vi "Dynamixel Motor Record and Playback Motion (Synchronous Write).vi"() -> ()   [LabVIEW 2016]
doc: "This example demonstrates how to capture sets of motor positions (frames) and then play them back. The playback feature also shows how to generate a sychronous write command that sets the goal position and velocity of all of the motors simultaneously."
uses:
  <instrlib>/Dynamixel Motor/Public/Motor Operation/Low Level/Baud Setting.ctl
  <instrlib>/Dynamixel Motor/Examples/Record And Playback Motion/Type Defs/Compiled Motion.ctl
  <instrlib>/Dynamixel Motor/Dynamixel Motor.lvlib
panel:
  in  "Initialize or Go":bool
  in  "Stop Playback":bool
  in  "Delay Time (ms)":dbl
  in  "Speed Scale (%)":dbl=100.0
  in  "Play":bool
  in  "Paste":bool
  in  "Copy":bool
  in  "Delete":bool
  in  "Insert":bool
  in  "Record":bool
  in  "Frame":u16
  in  "Step Time (ms)":u32=600
  in  "Baud rate (57600 bps)":T1=34 items=["1,000,000 bps"=1, "500,000 bps"=3, "400,000 bps"=4, "250,000 bps"=7, "200,000 bps"=9, "115200 bps"=16, "57600 bps"=34, "19200 bps"=103, "9600 bps"=207]
  in  "VISA resource name":refnum<visa-resource-name>
  in  "Up to":u8=253
  in  "From":u8
  in  "Refresh Motor List":bool
  in  "Motor Torques":cluster{"On":bool, "Off":bool, "ID":u8}[](array[cluster])
  in  "Torque off":bool
  in  "Save":bool
  in  "Load":bool
  in  "Quit":bool
  in  "Torque on":bool
  in  "Display Table":string[][](table)
  # "Motor List"
  # "Motor Torques"
  # "Frame number >>"
  # "Shortcuts: \n<Escape>-->Stop Playback\n<Enter>-->Go\n<Page Up>-->All on\n<Page Down>-->All off"
  # "1. Set the serial settings\n2. Run the VI\n3. click  Refresh Motor List to find connected motors.\n3. Click Record to capture the positions of all of the motors.\n4. Move the motors to a different position and click Record again.\n5. Change Frame to 0 or click on the first column of positions, then click Go.  Then Click Play.\n7. For more information and instructions, see the Readme."
  # "(c) 2011-2012  National Instruments.  ALL RIGHTS RESERVED."
  # "Playback"
  # "Record Positions"
  # "Initialization"
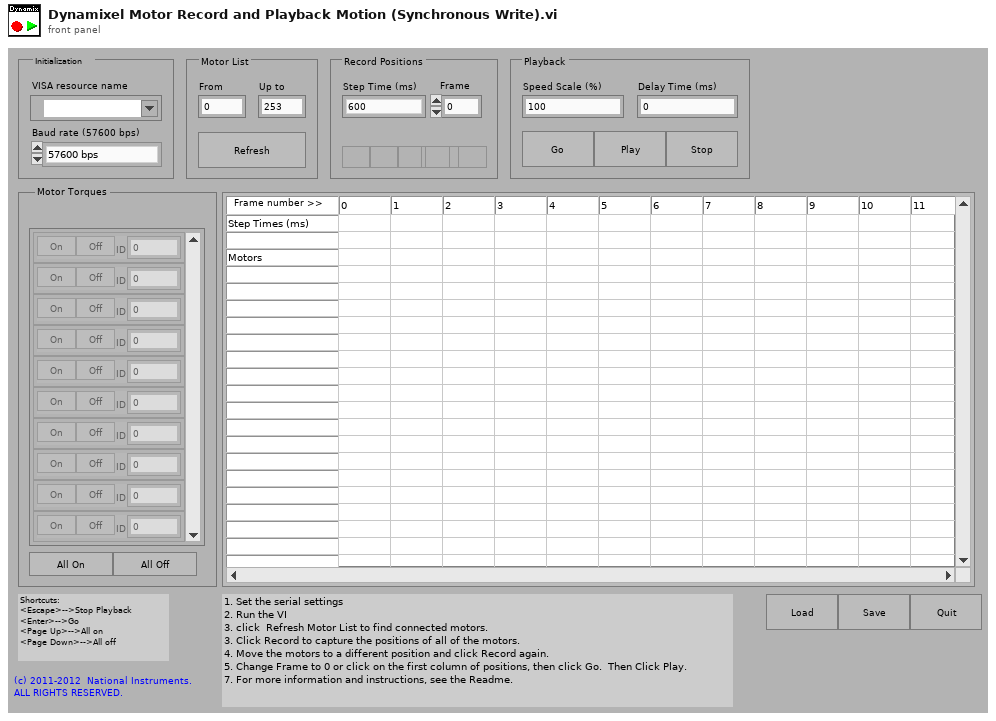
[diagram p1: front panel]
types:
  T1 = typedef "Dynamixel Motor.lvlib/Baud Setting.ctl" = u8
  T2 = typedef "Compiled Motion.ctl" = cluster{"Step Times":dbl[], "Serial Commands":string[], "Title":string}
  T3 = typedef "LVRowAndColumnTypeDef.ctl" = cluster{"Row":i32, "Column":i32}
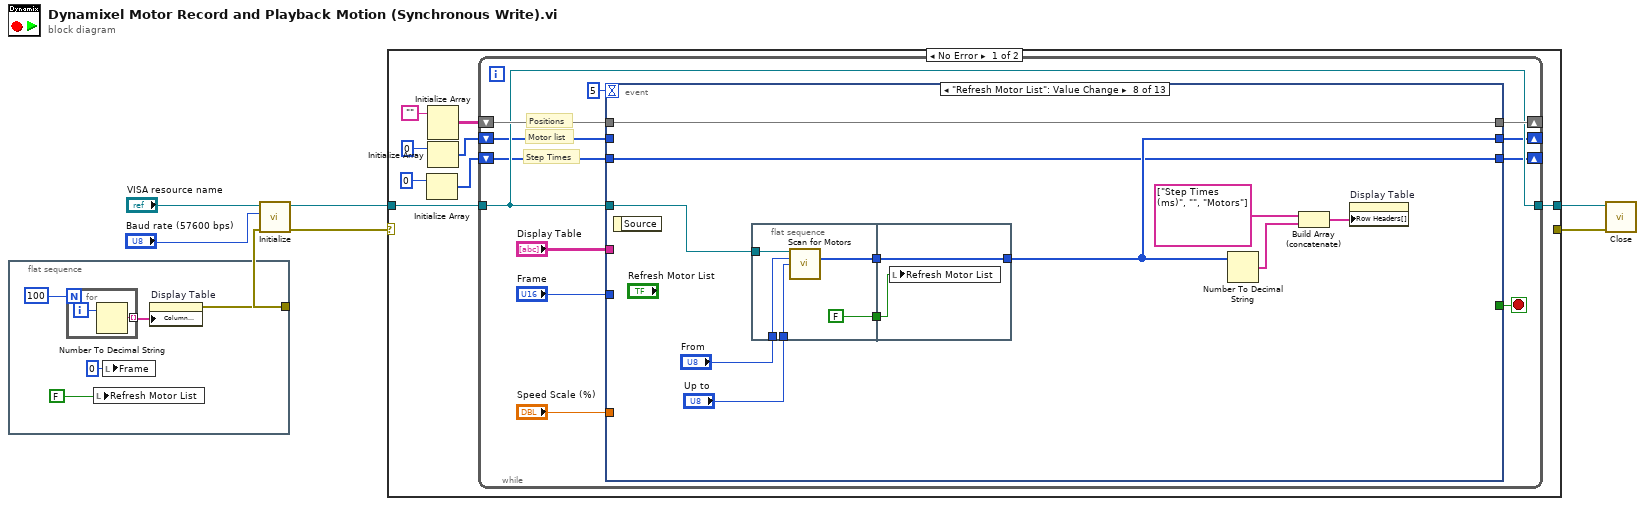
[diagram p0: block diagram]
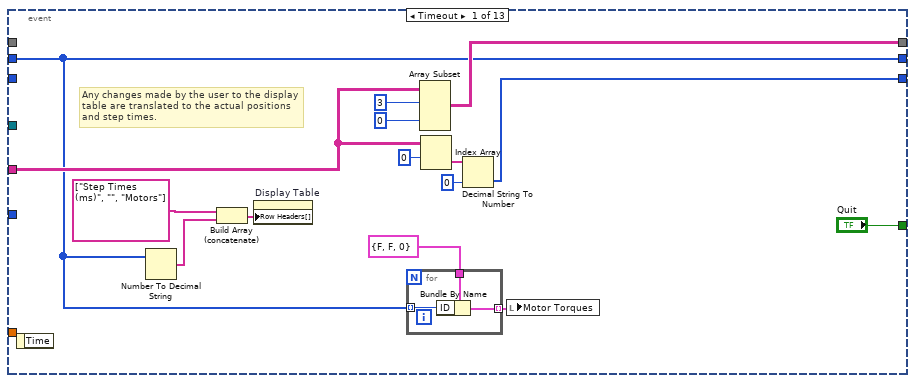
[diagram p2: hidden frame]
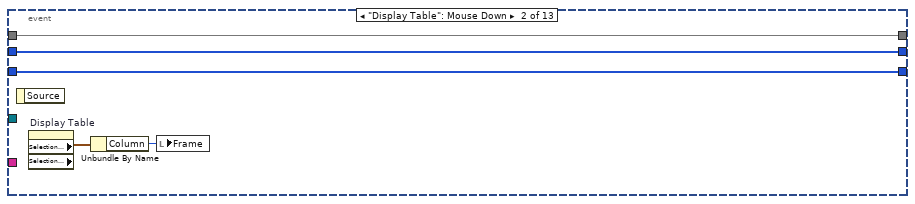
[diagram p3: hidden frame]
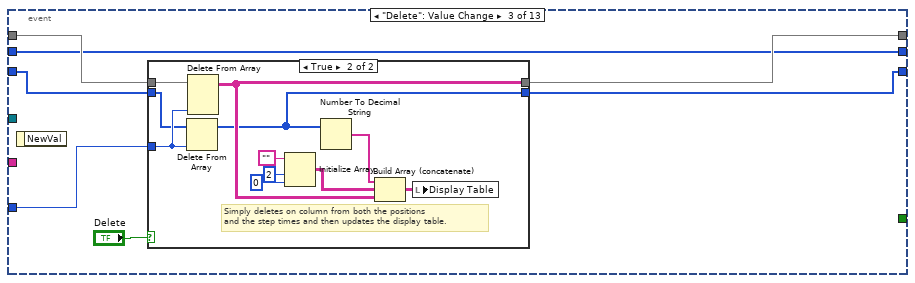
[diagram p4: hidden frame]
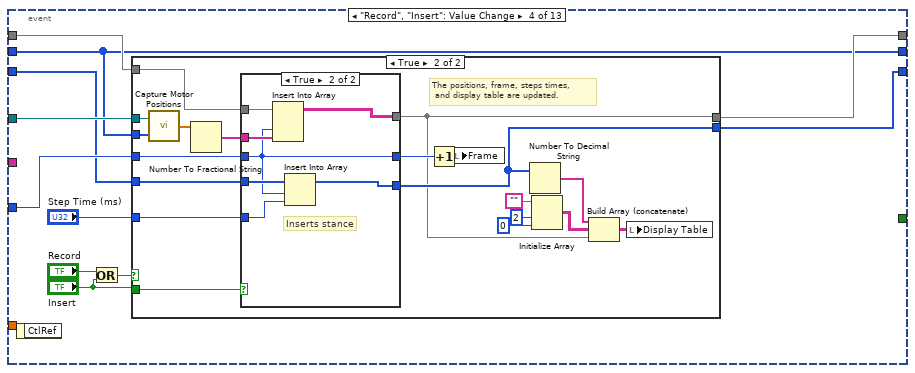
[diagram p6: hidden frame]
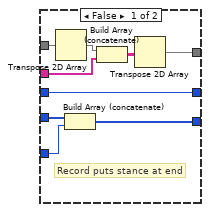
[diagram p8: hidden frame]
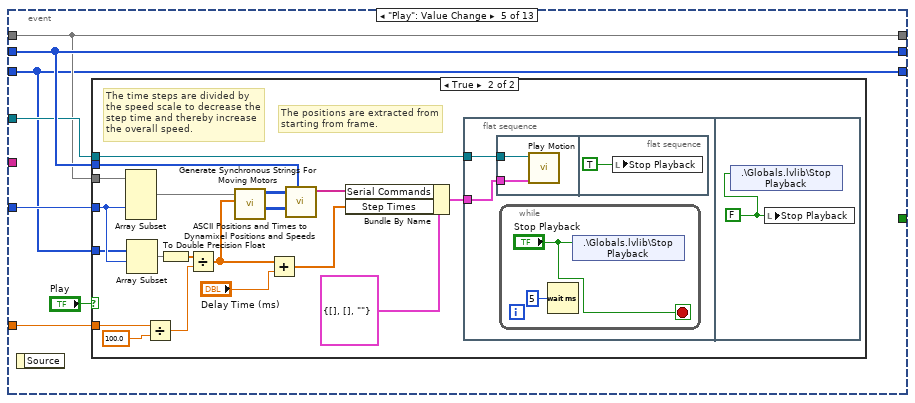
[diagram p9: hidden frame]
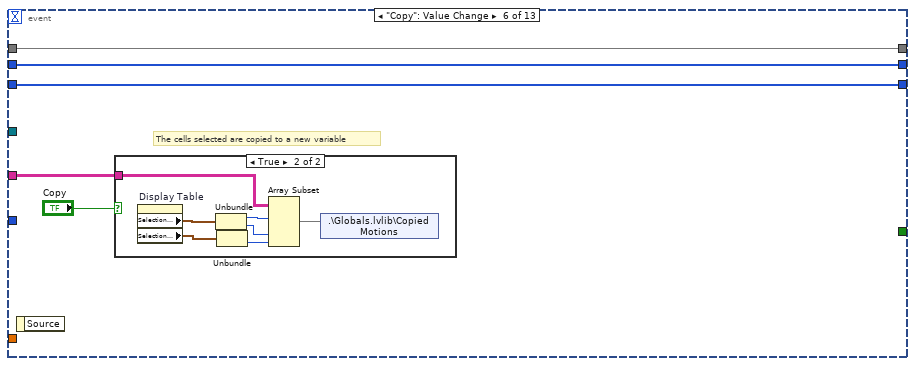
[diagram p11: hidden frame]
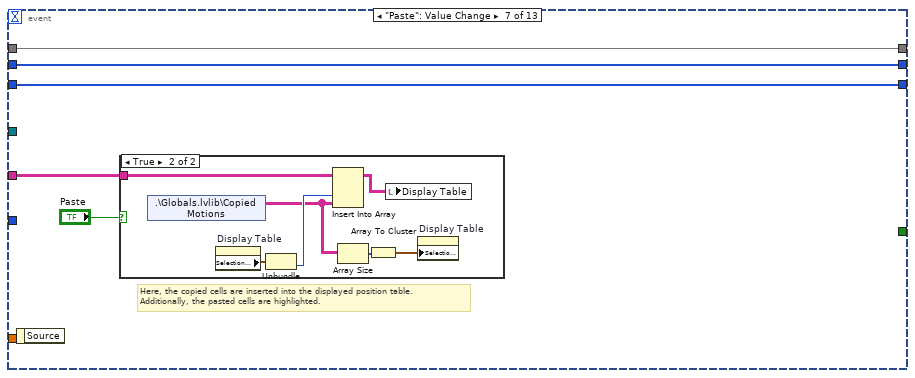
[diagram p13: hidden frame]
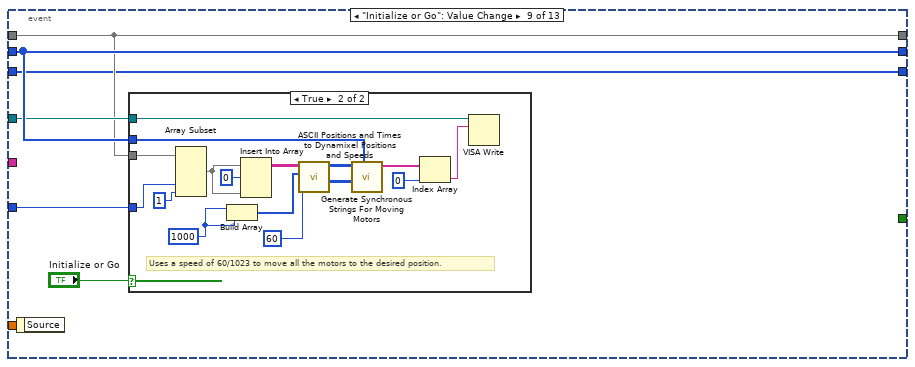
[diagram p15: hidden frame]
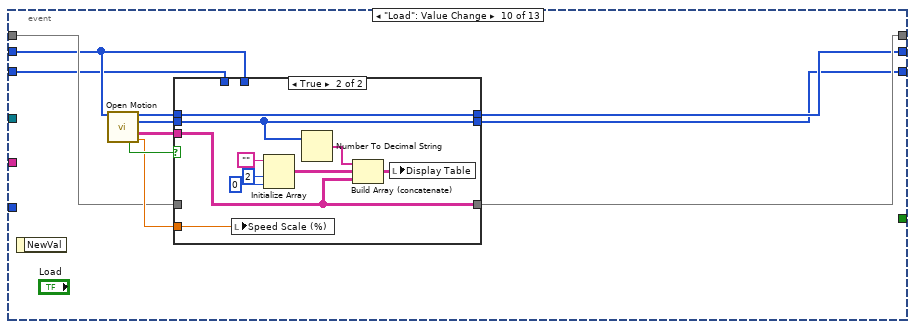
[diagram p17: hidden frame]
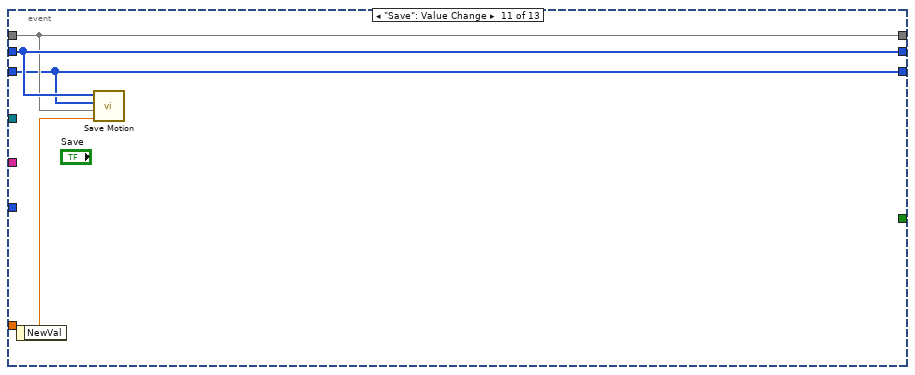
[diagram p19: hidden frame]
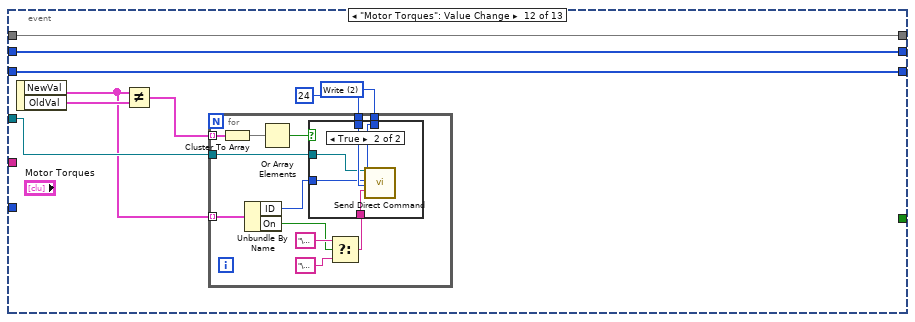
[diagram p20: hidden frame]
diagram:
  n1 = flat-sequence {
    tunnel: [w10] -> w4
    frame #0 {
      n2 = for {
        N: 100 -> [_]
        tunnel: [w13] -> w12 mode=indexing
        i -> [w14]
        n3 = Number To Decimal String(number=w14) -> (decimal integer string=w13:string)  [unwired: 1 in]
      }
      n4 = local write "Refresh Motor List"(FALSE ("Searching...")) -> ()
      n5 = local write "Frame"(u16 0 ("Frame")) -> ()
      n6 = property on="Display Table" class="Tbl (strict)"("Column Headers[]"=w12) -> (error out=w10:errorcluster)  [unwired: 2 in, 1 out]
    }
  }
  n7 = call <instrlib>:"Initialize.vi"("error in (no error)"=w4, "Baud rate (57600 bps)"="Baud rate (57600 bps)", "VISA resource name"="VISA resource name") -> ("error out"=w1:errorcluster, "VISA resource name out"=w7:refnum<visa-resource-name>)  [unwired: 7 in]
  n8 = case shown="No Error" w1 {
    selector: w1 -> [_ w290]
    tunnel: w7 -> [w22 w289]
    tunnel: [_ w290] -> w3
    tunnel: [w19 w289] -> w2
    frame No Error {
      n9 = Initialize Array(u32 0) -> (w15:u32[])  [unwired: 1 in]
      n10 = Initialize Array("") -> (w20:string[][])  [unwired: 2 in]
      n11 = Initialize Array(u8 0) -> (w18:u8[])  [unwired: 1 in]
      n12 = while {
        tunnel: w22 -> [w27]
        shift-right: [w29] -> _
        shift-left: w20 -> [w28]
        tunnel: [w27] -> w19
        shift-right: [w26] -> _
        shift-left: w18 -> [w25]
        shift-right: [w24] -> _
        shift-left: w15 -> [w23]
        stop <- w34 stop-if-true
        # "Step Times"
        # "Motor list"
        # "Positions"
        n13 = event shown="[7] \"Refresh Motor List\": Value Change" {
          selector: _ -> [_ _ _ _ _ _ _ _ _ _ _ _ _]
          dyn-events: _ -> [_ _ _ _ _ _ _ _ _ _ _ _ _]
          timeout: 5 -> [_ _ _ _ _ _ _ _ _ _ _ _ _]
          tunnel: "Frame" -> [_ _ w62 w84 w131 _ _ _ w206 _ _ _ _]
          tunnel: w27 -> [_ _ _ w83 w129 _ _ w191 w204 _ _ w256 w281]
          tunnel: w25 -> [w36 w54 w60 w80 w130 w161 w173 _ w205 w226 w251 w253 w279]
          tunnel: "Display Table" -> [w43 _ _ _ _ w164 w176 _ _ _ _ _ _]
          tunnel: w28 -> [_ w55 w63 w82 w127 w162 w174 w186 w203 w228 w249 w254 w280]
          tunnel: "Speed Scale (%)" -> [_ _ _ _ w128 _ _ _ _ _ w250 _ _]
          tunnel: ["Quit" _ _ _ _ _ _ _ _ _ _ _ _] -> w34
          tunnel: [w37 w55 w61 w81 w127 w162 w174 w186 w203 w229 w249 w254 w280] -> w29
          tunnel: [w36 w54 w60 w80 w130 w161 w173 w185 w205 w227 w251 w253 w279] -> w26
          tunnel: [w35 w53 w59 w79 w126 w160 w172 w184 w202 w225 w248 w252 w278] -> w24
          tunnel: w23 -> [_ w53 w58 w78 w126 w160 w172 w184 w202 w224 w248 w252 w278]
          event Timeout {
            # "Any changes made by the user to the display \ntable are translated to the actual positions \nand step times."
            n14 = event-data() -> ()  [unwired: 1 in, 1 out]
            n15 = Number To Decimal String(number=w36) -> (decimal integer string=w47:string[])  [unwired: 1 in]
            n16 = Build Array (concatenate)(string[] ["Step Times (ms)", "", "Motors"], w47) -> (w46:string[])
            n17 = property on="Display Table" class="Tbl (strict)"("Row Headers[]"=w46) -> ()  [unwired: 2 in, 2 out]
            n18 = for {
              tunnel: w36 -> [w52] mode=indexing
              tunnel: cluster{"On":bool, "Off":bool, "ID":u8} {"On"=FALSE, "Off"=FALSE, "ID"=0} ("Cluster") -> [w51]
              tunnel: [w50] -> w39 mode=indexing
              n19 = Bundle By Name(cluster=w51, "ID"=w52) -> (w50:cluster{"On":bool, "Off":bool, "ID":u8})
            }
            n20 = Array Subset(array=w43, index (row)=3 ("index"), index (col)=0 ("index")) -> (w37:string[][])  [unwired: 2 in]
            n21 = Index Array(array=w43, index (row)=0) -> (element=w42:string[])  [unwired: 1 in]
            n22 = Decimal String To Number(string=w42, default (0L)=u32 0 ("default (0 I32)")) -> (number=w35:u32[])  [unwired: 1 in, 1 out]
            n23 = local write "Motor Torques"(w39) -> ()
          }
          event "Display Table": Mouse Down {
            n24 = event-data() -> ()  [unwired: 1 in, 1 out]
            n25 = property on="Display Table" class="Tbl (strict)" props=["Selection Start", "Selection Size"]() -> ("Selection Start"=w57:T3)  [unwired: 2 in, 3 out]
            n26 = Unbundle By Name(w57) -> ("Column"=w56:i32)
            n27 = local write "Frame"(w56) -> ()
          }
          event "Delete": Value Change {
            n28 = event-data() -> ()  [unwired: 1 in, 1 out]
            n29 = case shown="True" "Delete" {
              tunnel: w62 -> [_ w70]
              tunnel: w63 -> [w66 w71]
              tunnel: [w66 w69] -> w61
              tunnel: [w65 w68] -> w59
              tunnel: w58 -> [w65 w67]
              frame False {
              }
              frame True {
                # "Simply deletes on column from both the positions \nand the step times and then updates the display table."
                n30 = Delete From Array(array=w67, index=w70) -> (array with subset deleted=w68:u32[])  [unwired: 1 in, 1 out]
                n31 = Delete From Array(array=w71, index (col)=w70) -> (array with subset deleted=w69:string[][])  [unwired: 2 in, 1 out]
                n32 = Initialize Array("", 2 ("dimension size"), 0 ("dimension size")) -> (w74:string[][])
                n33 = Number To Decimal String(number=w68) -> (decimal integer string=w77:string[])  [unwired: 1 in]
                n34 = Build Array (concatenate)(w77, w74, w69) -> (w73:string[][])
                n35 = local write "Display Table"(w73) -> ()
              }
            }
          }
          event "Record", "Insert": Value Change {
            n36 = event-data() -> ()  [unwired: 1 in, 1 out]
            n37 = Or(x="Record", y="Insert") -> (x .or. y?=w87:bool)
            n38 = case shown="True" w87 {
              tunnel: w83 -> [_ w109]
              tunnel: "Insert" -> [_ w108]
              tunnel: w82 -> [w90 w106]
              tunnel: w80 -> [_ w105]
              tunnel: w84 -> [_ w95]
              tunnel: "Step Time (ms)" -> [_ w92]
              tunnel: [w90 w91] -> w81
              tunnel: [w89 w94] -> w79
              tunnel: w78 -> [w89 w93]
              frame False {
              }
              frame True {
                # "The positions, frame, steps times,\n and display table are updated."
                n39 = call <instrlib>:"Capture Motor Positions.vi"("Motor List (Numeric)"=w105, "Com Port"=w109) -> ("Positions (deg)"=w97:dbl[])
                n40 = Number To Fractional String(number=w97) -> (F-format string=w107:string[])  [unwired: 3 in]
                n41 = case shown="True" w108 {
                  tunnel: w106 -> [w117 w125]
                  tunnel: w107 -> [w115 w124]
                  tunnel: w95 -> [w118 w121]
                  tunnel: [w113 w123] -> w91
                  tunnel: [w118 w121] -> w96
                  tunnel: w93 -> [w111 w122]
                  tunnel: w92 -> [w112 w120]
                  tunnel: [w110 w119] -> w94
                  frame False {
                    # "Record puts stance at end"
                    n42 = Transpose 2D Array(2D array=w117) -> (transposed array=w116:string[][])
                    n43 = Build Array (concatenate)(w111, w112) -> (w110:u32[])
                    n44 = Build Array (concatenate)(w116, w115) -> (w114:string[][])
                    n45 = Transpose 2D Array(2D array=w114) -> (transposed array=w113:string[][])
                  }
                  frame True {
                    # "Inserts stance"
                    n46 = Insert Into Array(array=w125, index (col)=w121, new element=w124) -> (w123:string[][])  [unwired: 1 in]
                    n47 = Insert Into Array(array=w122, index=w121, new element=w120) -> (w119:u32[])
                  }
                }
                n48 = Increment(x=w96) -> (x+1=w104:u16)
                n49 = local write "Frame"(w104) -> ()
                n50 = Number To Decimal String(number=w94) -> (decimal integer string=w98:string[])  [unwired: 1 in]
                n51 = Initialize Array("", 2 ("dimension size"), 0 ("dimension size")) -> (w101:string[][])
                n52 = Build Array (concatenate)(w98, w101, w91) -> (w102:string[][])
                n53 = local write "Display Table"(w102) -> ()
              }
            }
          }
          event "Play": Value Change {
            n54 = event-data() -> ()  [unwired: 1 in, 1 out]
            n55 = case shown="True" "Play" {
              tunnel: w131 -> [_ w148]
              tunnel: w126 -> [_ w147]
              tunnel: w127 -> [_ w146]
              tunnel: w130 -> [_ w138]
              tunnel: w129 -> [_ w145]
              tunnel: w128 -> [_ w144]
              frame False {
              }
              frame True {
                # "The positions are extracted from \nstarting from frame."
                # "The time steps are divided by \nthe speed scale to decrease the \nstep time and thereby increase \nthe overall speed."
                n56 = Array Subset(array=w146, index (col)=w148) -> (w140:string[][])  [unwired: 3 in]
                n57 = Array Subset(array=w147, index=w148) -> (w141:u32[])  [unwired: 1 in]
                n58 = Divide(x=w144, y=100.0) -> (x/y=w143:dbl)
                n59 = To Double Precision Float(number=w141) -> (double precision float=w133:dbl[])
                n60 = Divide(x=w133, y=w143) -> (x/y=w135:dbl[])
                n61 = call <instrlib>:"ASCII Positions and Times to Dynamixel Positions and Speeds.vi"("Step Times (ms)"=w135, "Positions"=w140) -> ("Dynamixel Speeds"=w134:u16[][], "Dynamixel Positions"=w139:u16[][])  [unwired: 8 in]
                n62 = Add(x=w135, y="Delay Time (ms)") -> (x+y=w150:dbl[])
                n63 = call <instrlib>:"Generate Synchronous Strings For Moving Motors.vi"("Motor List"=w138, "Dynamixel Speeds"=w134, "Dynamixel Positions"=w139) -> ("Compiled Sync Parameters"=w137:string[])  [unwired: 7 in, 1 out]
                n64 = Bundle By Name(cluster=T2 {"Step Times"=[], "Serial Commands"=[], "Title"=""} ("Play Gait"), "Serial Commands"=w137, "Step Times"=w150) -> (w149:T2)
                n65 = flat-sequence {
                  tunnel: w149 -> [w153]
                  tunnel: w145 -> [w152]
                  frame #0 {
                    n66 = flat-sequence {
                      tunnel: w153 -> [w155]
                      tunnel: w152 -> [w154]
                      frame #0 {
                        n67 = call <instrlib>:"Play Motion.vi"("Compiled motion"=w155, "Com Port"=w154) -> ()  [unwired: 9 in, 1 out]
                      }
                      frame #1 {
                        n68 = local write "Stop Playback"(TRUE ("Stop Play")) -> ()
                      }
                    }
                    n69 = while {
                      stop <- "Stop Playback" stop-if-true
                      n70 = Wait (ms)(milliseconds to wait=u32 5) -> ()  [unwired: 1 out]
                      n71 = shared-variable ".\\Globals.lvlib\\Stop Playback"("Stop Playback") -> ()  [unwired: 1 in, 1 out]
                    }
                  }
                  frame #1 {
                    w159 = FALSE ("Stop Play")
                    n72 = shared-variable ".\\Globals.lvlib\\Stop Playback"(w159) -> ()  [unwired: 1 in, 1 out]
                    n73 = local write "Stop Playback"(w159) -> ()
                  }
                }
              }
            }
          }
          event "Copy": Value Change {
            # "The cells selected are copied to a new variable"
            n74 = event-data() -> ()  [unwired: 1 in, 1 out]
            n75 = case shown="True" "Copy" {
              tunnel: w164 -> [_ w166]
              frame False {
              }
              frame True {
                n76 = property on="Display Table" class="Tbl (strict)"() -> ("Selection Start"=w171:T3, "Selection Size"=w170:T3)  [unwired: 2 in, 2 out]
                n77 = Unbundle(w171) -> ("Row"=w169:i32, "Column"=w168:i32)
                n78 = Unbundle(w170) -> ("Column"=w167:i32)  [unwired: 1 out]
                n79 = Array Subset(array=w166, index (row)=w169, index (col)=w168, length (col)=w167) -> (w165:string[][])  [unwired: 1 in]
                n80 = shared-variable ".\\Globals.lvlib\\Copied Motions"(w165) -> ()  [unwired: 1 in, 1 out]
              }
            }
          }
          event "Paste": Value Change {
            # "Here, the copied cells are inserted into the displayed position table.  \nAdditionally, the pasted cells are highlighted."
            n81 = event-data() -> ()  [unwired: 1 in, 1 out]
            n82 = case shown="True" "Paste" {
              tunnel: w176 -> [_ w178]
              frame False {
              }
              frame True {
                n83 = shared-variable ".\\Globals.lvlib\\Copied Motions"() -> (w177:string[][])  [unwired: 1 in, 1 out]
                n84 = property on="Display Table" class="Tbl (strict)"() -> ("Selection Start"=w183:T3)  [unwired: 2 in, 2 out]
                n85 = Unbundle(w183) -> ("Column"=w182:i32)  [unwired: 1 out]
                n86 = Insert Into Array(array=w178, index (col)=w182, new element=w177) -> (w181:string[][])  [unwired: 1 in]
                n87 = Array Size(array=w177) -> (size(s)=w180:i32[])
                n88 = Array To Cluster(array=w180) -> (cluster=w179:cluster{"[0]":i32, "[1]":i32})
                n89 = local write "Display Table"(w181) -> ()
                n90 = property on="Display Table" class="Tbl (strict)"("Selection Size"=w179) -> ()  [unwired: 2 in, 2 out]
              }
            }
          }
          event "Refresh Motor List": Value Change {
            n91 = event-data() -> ()  [unwired: 1 in, 1 out]
            n92 = flat-sequence {
              tunnel: [w198] -> w190
              tunnel: [FALSE ("Searching...")] -> w189
              tunnel: "Up to" -> [w196]
              tunnel: "From" -> [w195]
              tunnel: w191 -> [w199]
              tunnel: [w201] -> w185
              tunnel: w190 -> [w201]
              tunnel: w189 -> [w200]
              frame #0 {
                n93 = call <instrlib>:"Scan for Motors.vi"("VISA resource name"=w199, "Starting ID (0)"=w195, "Ending ID (253)"=w196) -> ("Motors IDs Found"=w198:u8[])  [unwired: 10 in, 2 out]
              }
              frame #1 {
                n94 = local write "Refresh Motor List"(w200) -> ()
              }
            }
            n95 = Number To Decimal String(number=w185) -> (decimal integer string=w194:string[])  [unwired: 1 in]
            n96 = Build Array (concatenate)(string[] ["Step Times (ms)", "", "Motors"], w194) -> (w192:string[])
            n97 = property on="Display Table" class="Tbl (strict)"("Row Headers[]"=w192) -> ()  [unwired: 2 in, 2 out]
          }
          event "Initialize or Go": Value Change {
            n98 = event-data() -> ()  [unwired: 1 in, 1 out]
            n99 = case shown="True" "Initialize or Go" {
              tunnel: w203 -> [_ w218]
              tunnel: w206 -> [_ w217]
              tunnel: w205 -> [_ w210]
              tunnel: w204 -> [_ w216]
              frame False {
              }
              frame True {
                w215 = 1000
                # "Uses a speed of 60/1023 to move all the motors to the desired position."
                n100 = Array Subset(array=w218, index (col)=w217, length (col)=1) -> (w222:string[][])  [unwired: 2 in]
                n101 = Build Array(w215, w215) -> (w213:i32[])
                n102 = Insert Into Array(array=w222, index (col)=0, new element=w222) -> (w214:string[][])  [unwired: 1 in]
                n103 = call <instrlib>:"ASCII Positions and Times to Dynamixel Positions and Speeds.vi"("Minimum Speed (Max RPM)"=60, "Step Times (ms)"=w213, "Positions"=w214) -> ("Dynamixel Speeds"=w208:u16[][], "Dynamixel Positions"=w211:u16[][])  [unwired: 7 in]
                n104 = call <instrlib>:"Generate Synchronous Strings For Moving Motors.vi"("Motor List"=w210, "Dynamixel Speeds"=w208, "Dynamixel Positions"=w211) -> ("Compiled Sync Parameters"=w209:string[])  [unwired: 7 in, 1 out]
                n105 = Index Array(array=w209, index=0) -> (element=w219:string)
                n106 = VISA Write(VISA resource name=w216, write buffer=w219) -> ()  [unwired: 1 in, 3 out]
              }
            }
          }
          event "Load": Value Change {
            n107 = event-data() -> ()  [unwired: 1 in, 1 out]
            n108 = call <instrlib>:"Open Motion.vi"("Motor List In"=w226) -> ("Motor List"=w234:u8[], "Motion times"=w233:u32[], "Motion Positions"=w232:string[][], "File found?"=w231:bool, "Speed Scale"=w230:dbl)  [unwired: 10 in]
            n109 = case shown="True" w231 {
              tunnel: w234 -> [_ w239]
              tunnel: w233 -> [_ w238]
              tunnel: w232 -> [_ w240]
              tunnel: w230 -> [_ w241]
              tunnel: [w237 w240] -> w229
              tunnel: w228 -> [w237 _]
              tunnel: [w236 w239] -> w227
              tunnel: w226 -> [w236 _]
              tunnel: [w235 w238] -> w225
              tunnel: w224 -> [w235 _]
              frame False {
              }
              frame True {
                n110 = local write "Speed Scale (%)"(w241) -> ()
                n111 = Initialize Array("", 2 ("dimension size"), 0 ("dimension size")) -> (w244:string[][])
                n112 = Number To Decimal String(number=w238) -> (decimal integer string=w247:string[])  [unwired: 1 in]
                n113 = Build Array (concatenate)(w247, w244, w240) -> (w243:string[][])
                n114 = local write "Display Table"(w243) -> ()
              }
            }
          }
          event "Save": Value Change {
            n115 = event-data() -> ()  [unwired: 1 in, 1 out]
            n116 = call <instrlib>:"Save Motion.vi"("Speed Scale"=w250, "Positions"=w249, "Step Times"=w248, "Motor List"=w251) -> ()  [unwired: 8 in]
          }
          event "Motor Torques": Value Change {
            w259 = u16 2 items=["Ping", "Read", "Write", "Registered Write", "Action", "Reset", "Sync Write"] ("Select Action")
            n117 = event-data() -> ("NewVal"=w255:cluster{"On":bool, "Off":bool, "ID":u8}[], "OldVal"=w257:cluster{"On":bool, "Off":bool, "ID":u8}[])  [unwired: 1 in]
            n118 = Not Equal?(x=w255, y=w257) -> (x != y?=w260:cluster{"On":bool, "Off":bool, "ID":bool}[])
            n119 = for {
              tunnel: w260 -> [w267] mode=indexing
              tunnel: w259 -> [w270]
              tunnel: u8 24 ("Address") -> [w264]
              tunnel: w256 -> [w263]
              tunnel: w255 -> [w262] mode=indexing
              n120 = Cluster To Array(cluster=w267) -> (array=w272:bool[])
              n121 = Unbundle By Name(w262) -> ("ID"=w261:u8, "On"=w266:bool)
              n122 = Or Array Elements(Boolean array=w272) -> (logical OR=w271:bool)
              n123 = Select(t="\u0001", s=w266, f="\u0000") -> (s? t:f=w265:string)
              n124 = case shown="True" w271 {
                tunnel: w270 -> [_ w277]
                tunnel: w265 -> [_ w276]
                tunnel: w264 -> [_ w275]
                tunnel: w263 -> [_ w274]
                tunnel: w261 -> [_ w273]
                frame False {
                }
                frame True {
                  n125 = call <instrlib>:"Send Direct Command.vi"("VISA resource name"=w274, "Select Action"=w277, "Motor ID (0)"=w273, "Address"=w275, "Parameters"=w276) -> ()  [unwired: 12 in, 3 out]
                }
              }
            }
          }
          event "Torque on", "Torque off": Value Change {
            w284 = u16 2 items=["Ping", "Read", "Write", "Registered Write", "Action", "Reset", "Sync Write"] ("Select Action")
            n126 = event-data() -> ()  [unwired: 1 in, 1 out]
            n127 = Select(t="\u0001", s="Torque on", f="\u0000") -> (s? t:f=w286:string)
            n128 = call <instrlib>:"Send Direct Command.vi"("VISA resource name"=w281, "Select Action"=w284, "Motor ID (0)"=u8 254 ("Motor ID"), "Address"=u8 24, "Parameters"=w286) -> ()  [unwired: 12 in, 3 out]
          }
        }
      }
    }
    frame Error {
    }
  }
  n129 = call <instrlib>:"Close.vi"("error in (no error)"=w3, "VISA resource name"=w2) -> ()  [unwired: 9 in, 1 out]
